vi "Complex.vi"() -> (0 "error out":errorcluster, 3 "Passed?":bool)   [LabVIEW 2009]
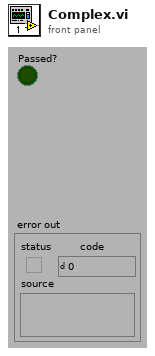
[diagram p1: front panel]
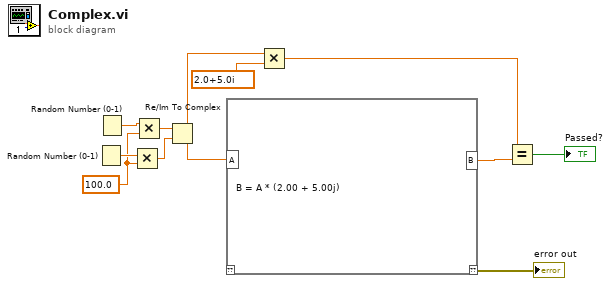
[diagram p0: block diagram]
diagram:
  w5 = 100.0 ("y")
  n1 = Random Number (0-1)() -> (number: 0 to 1=w10:dbl)
  n2 = Random Number (0-1)() -> (number: 0 to 1=w6:dbl)
  n3 = Multiply(x=w10, y=w5) -> (x*y=w4:dbl)
  n4 = Multiply(x=w6, y=w5) -> (x*y=w7:dbl)
  n5 = Re/Im To Complex(1:w4, 2:w7) -> (0:w3:cdb)
  n6 = script code="B = A * (2.00 + 5.00j)"("A"=w3) -> ("??"=→"error out":errorcluster, "B"=w9:cdb)  [unwired: 1 in]
  n7 = Multiply(x=w3, y=cdb 2.0+5.0i) -> (x*y=w1:cdb)
  n8 = Equal?(x=w1, y=w9) -> (x = y?=→"Passed?":bool)
